vi "get_data.vi"(11 "SquareTeam.lvlib:MyTeam.lvclass":refnum<class "MyTeam.lvclass">) -> (2 "center of mass":dbl[](array[numeric]), 3 "map":T1[][](array[typedef]))   [LabVIEW 2020, in "The_Hill_Youth.lvlib" / "MyTeam.lvclass"]
uses:
  MyTeam.lvclass
  map_point.ctl
  MyTeam.lvclass/MyTeam.ctl
  The_Hill_Youth.lvlib
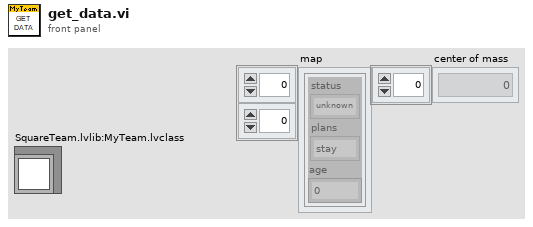
[diagram p1: front panel]
types:
  T1 = typedef "The_Hill_Youth.lvlib/map_point.ctl" = cluster{"status":enum16{"unknown", "frind", "enemy", "empty"}, "plans":enum16{"stay", "duplicate", "attack", "move to", "no plans"}, "age":dbl}
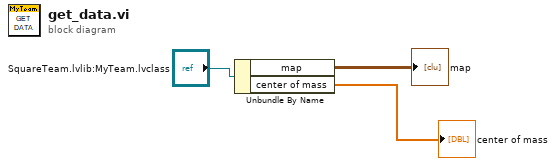
[diagram p0: block diagram]
diagram:
  n1 = Unbundle By Name("SquareTeam.lvlib:MyTeam.lvclass") -> ("map"=→"map":T1[][], "center of mass"=→"center of mass":dbl[])
